vi "OpenCreateVI.vi"(8 "error in":errorcluster, 11 "State":T1) -> (0 "error out":errorcluster, 3 "State out":T1)   [LabVIEW 2013, in "data interface script.lvlib"]
uses:
  data interface script.lvlib
  Controls/StateCluster.ctl
  Controls/initialized references.ctl
  Controls/interface VI type.ctl
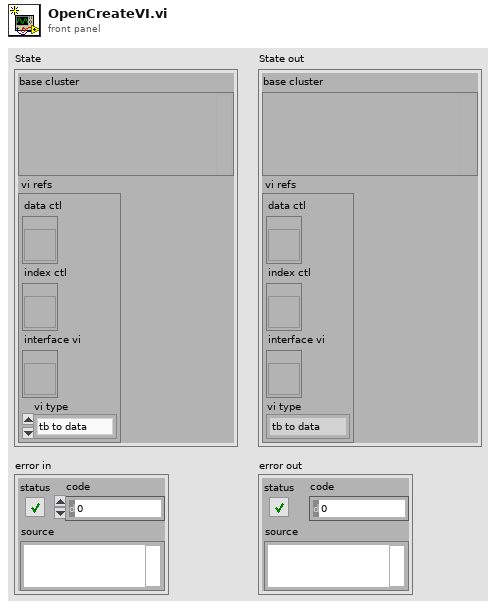
[diagram p1: front panel]
types:
  T1 = typedef "data interface script.lvlib/StateCluster.ctl" = cluster{"base cluster":variant, "vi refs":T2}
  T2 = typedef "data interface script.lvlib/initialized references.ctl" = cluster{"data ctl":refnum<vi>, "index ctl":refnum<vi>, "interface vi":refnum<vi>, "vi type":T3}
  T3 = typedef "data interface script.lvlib/interface VI type.ctl" = enum16{"tb to data", "data to tb"}
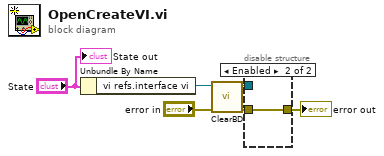
[diagram p0: block diagram]
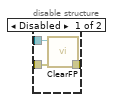
[diagram p2: hidden frame]
diagram:
  n1 = Unbundle By Name("State") -> ("vi refs.interface vi"=w2:refnum<vi>)
  n2 = call "ClearBD.vi"("error in"="error in", "reference"=w2) -> ("error out"=w6:errorcluster, "reference out"=w5:refnum<vi>)  [unwired: 8 in]
  n3 = disable-structure shown="Enabled" {
    disable-tunnel: w6 -> [w9 w10]
    disable-tunnel: w5 -> [w8 _]
    disable-tunnel: [w7 w10] -> w1
    frame Disabled {
      n4 = call "ClearFP.vi"("error in"=w9, "reference"=w8) -> ("error out"=w7:errorcluster)  [unwired: 8 in, 1 out]
    }
    frame Enabled {
    }
  }
  "error out" <- w1
  "State out" <- "State"
